vi "GUI Main Window.vi"() -> ()   [LabVIEW 2011]
doc: "Fast Orbit Feedback (FOFB) graphical user interface."
uses:
  Types Definitions/Type Configuration Loop Mode.ctl
  <vilib>/Platform/TimedLoop/XDataNode/timing_clust.ctl
  <vilib>/Platform/TimedLoop/XDataNode/nitl_modes.ctl
  <vilib>/Platform/TimedLoop/XDataNode/wakeup.ctl
  Types Definitions/Type Diagnostics Sample.ctl
  Types Definitions/Type Diagnostics Data.ctl
  Types Definitions/Type CPU Loads Array.ctl
  Types Definitions/Type CPU Loads.ctl
  Types Definitions/Type Monitoring Sample.ctl
  Types Definitions/Type FOFB Parameters.ctl
  Types Definitions/Type Network Configuration.ctl
  Types Definitions/Type FA Configuration.ctl
  Types Definitions/Type Response Matrix Measurement Configuration.ctl
  Types Definitions/Type Correction Algorithm Configuration.ctl
  Types Definitions/Type Acquisition Network Configuration.ctl
  Types Definitions/Type Actuation Network Configuration.ctl
  Types Definitions/Type BPM or PS Selector.ctl
  <vilib>/Analysis/5stat.llb/RMS (DBL).vi
  GUI Monitoring Graph Selection Window.vi
  <vilib>/Platform/TimedLoop/XDataNode/XDataNode.xnode
  <vilib>/Platform/TimedLoop/XDataNode/XDNodeRunTimeDep.lvlib
  File VIs.lvlib
  Type Definitions.lvlib
  Third Party/bean/bean.lvlib
  User Interface Window VIs.lvlib
  User Interface VIs.lvlib
  XML VIs.lvlib
  Filter VIs.lvlib
  <vilib>/Analysis/NI_AALPro.lvlib
panel:
  out "error out":errorcluster
  out "Connected":bool
  in  "Open Computer Performance":bool
  in  "Open BPM RMS/Min/Max Monitoring Graph":bool
  out "Orbit Path":path caption="Endereço da Órbita de Referência"
  in  "Open Configuration GUI":bool
  in  "Max Scale Y":dbl=1.0 min=0.001 max=20.0 format="%6.3g"
  in  "Max Scale X":dbl=1.0 min=0.001 max=20.0 format="%6.3g"
  in  "Auto-Scale":bool
  in  "Open BPM-PS Monitoring Graph":bool
  out "Reference Orbit":dbl[](array[numeric])
  in  "Orbit Source":enum32{"Zero", "From File", "Current Orbit"}(radio)
  out "Current Orbit":dbl[](array[numeric])
  out "Operation Mode (Controller to GUI)":T1(ring) caption="Modo de Operação"
  in  "Send Orbit":bool
  out "Min Y @":string="AMP05A" caption="@"
  out "MaxY @":string="AMP05A" caption="@"
  out "RMS Y":dbl=-1.1111 caption="RMS =" format="%#.4g"
  out "Min Y":dbl=-1.2564 caption="Min =" format="%#.4g"
  out "Max. Y":dbl=1.1111 caption="Max =" format="%#.4g"
  out "Min X @":string="AMP01A" caption="@"
  out "Max X @":string="AMP01A" caption="@"
  out "RMS X":dbl=21.1111 caption="RMS =" format="%#.4g"
  out "Min X":dbl=1.1111 caption="Min =" format="%#.4g"
  out "Max. X":dbl=1.1111 caption="Max =" format="%#.4g"
  out "Horizontal":cluster{i32, dbl}[](graph)
  out "Vertical":cluster{i32, dbl}[](graph)
  in  "Save Orbit":bool
  # "Órbita de Referência Local"
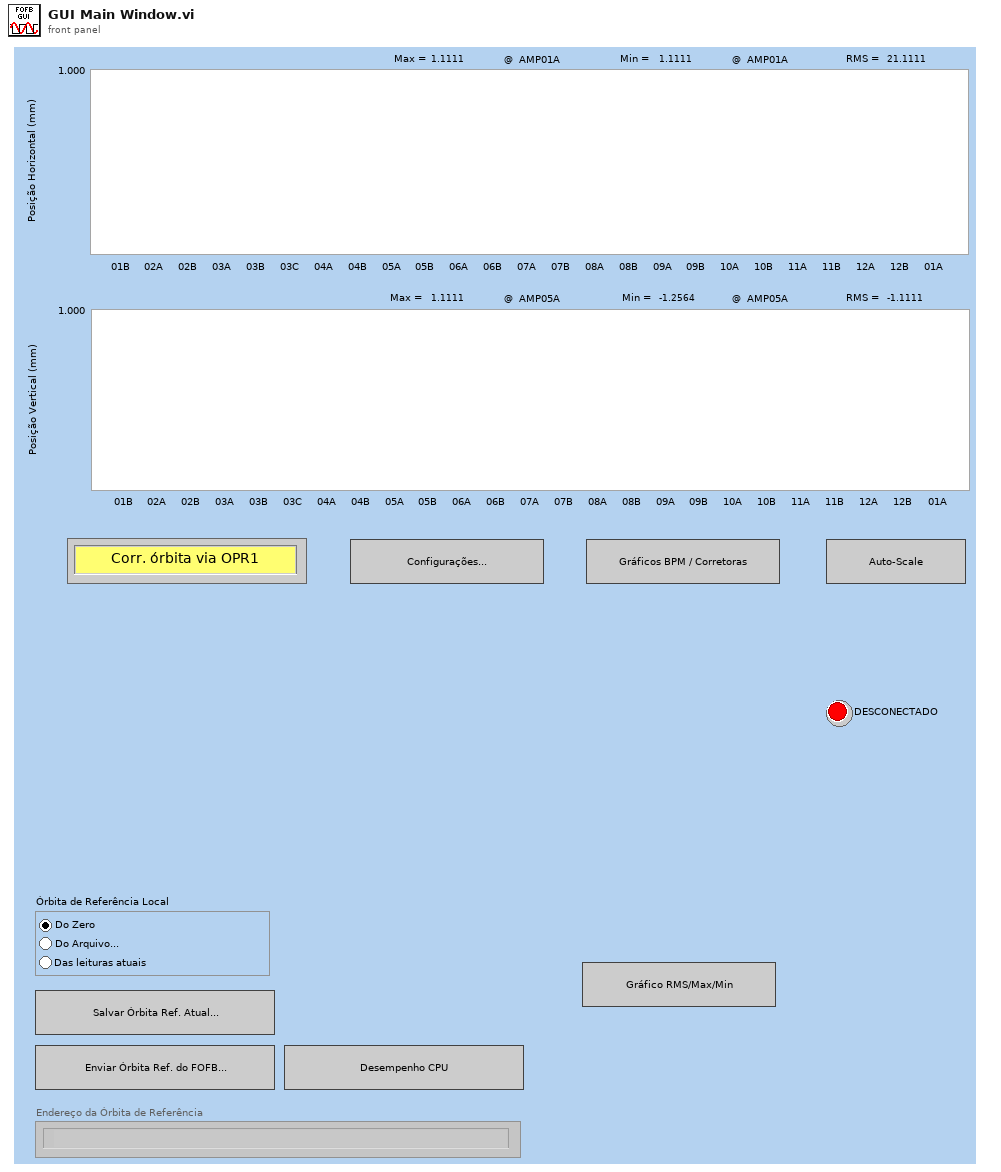
[diagram p1: front panel]
types:
  T1 = enum16{"Corr. órbita via OPR1", "Corr. órbita via FOFB", "Medida de Matriz Resposta"}
  T2 = enum8{"Enabled", "Disabled", "Disabled and Grayed Out"}
  T3 = typedef "Type Definitions.lvlib/Type Configuration Loop Mode.ctl" = enum8{"Operation Mode", "Request FOFB Parameters", "Send New FOFB Parameters", "Send Reference Orbit", "Request Response Matrix List Folder"}
  T4 = typedef "XDNodeRunTimeDep.lvlib/timing_clust.ctl" = cluster{"Expected End [f-1]":u64, "Actual End [f-1]":u64, "Finished Late? [f-1]":bool, "Expected End [i-1]":u64, "Actual End [i-1]":u64, "Finished Late? [i-1]":bool, "Expected Start [i]":u64, "Actual Start [i]":u64, "Expected Start [f]":u64, "Actual Start [f]":u64, "Source Name":string, "Structure Name":string, "Period":i64, "Deadline":i64, "Offset":i64, "Start":i64, "Priority":i32, "Timeout":i32, "Mode":T5, "Wakeup Reason":T6, "Error":errorcluster, "Source Type":string, "Secondary Source Type":string, "Global End Time":u64, "Global Start Time":u64, "Frame Duration":u64, "Iteration Duration":u64, "Assigned CPU":i32, "I/O Scan Engine Mode":u32}
  T5 = typedef "XDNodeRunTimeDep.lvlib/nitl_modes.ctl" = enum32{"No Change", "Process missed periods, maintain original phase", "Discard missed periods, maintain original phase", "Process missed periods, ignore original phase", "Discard missed periods, ignore original phase"}
  T6 = typedef "XDNodeRunTimeDep.lvlib/wakeup.ctl" = enum32{"Normal", "Aborted", "Asynchronous wakeup", "Timing source error", "Timed loop error", "Timeout"}
  T7 = enum32{"Invalid", "Standard", "Closed", "Hidden", "Minimized", "Maximized"}
  T8 = typedef "Type Definitions.lvlib/Type BPM or PS Selector.ctl" = cluster{"Name":string, "Active":bool}
  T9 = typedef "Type Definitions.lvlib/Type Diagnostics Sample.ctl" = cluster{"Timestamp":timestamp, "Diagnostics Data":T10}
  T10 = typedef "Type Definitions.lvlib/Type Diagnostics Data.ctl" = cluster{"Time-Critical Loop Missed Iterations":u32, "Time-Critical Loop Execution Time (usec)":u32, "FA Buffer Usage":u32, "Available Memory (bytes)":u32, "CPU Loads Array":T11}
  T11 = typedef "Type Definitions.lvlib/Type CPU Loads Array.ctl" = T12[]
  T12 = typedef "Type Definitions.lvlib/Type CPU Loads.ctl" = cluster{"Total (%)":dbl, "Time Critical (%)":dbl, "Timed Structures (%)":dbl, "High (%)":dbl, "Above Normal (%)":dbl, "Normal (%)":dbl, "Background (%)":dbl, "Idle (%)":dbl, "ISR (%)":dbl}
  T13 = enum16{"open", "open or create", "create or replace", "create", "open (read-only)"}
  T14 = typedef "Type Definitions.lvlib/Type FOFB GUI.ctl" = cluster{"Response Matrix List Folder Notifier":refnum<notifier>, "Send Reference Orbit Notifier":refnum<notifier>, "FOFB Parameters Notifier":refnum<notifier>, "Configuration Loop Mode Notifier":refnum<notifier>, "Stop VIs Notifier":refnum<notifier>, "GUI Configuration Notifier":refnum<notifier>, "Monitoring Data Notifier":refnum<queue>, "Performance Monitoring Data Notifier":refnum<queue>, "BPM / PS Monitoring Data Notifiers":refnum<queue>[], "Load Orbit Notifier":refnum<notifier>, "RMS Monitoring Data Queue":refnum<queue>, "GUI-Controller Connected Queue":refnum<queue>}
  T15 = typedef "Type Definitions.lvlib/Type FOFB Parameters.ctl" = cluster{"Network":T16, "Fast Acquisition":T17, "Response Matrix Measurement":T18, "Correction Algorithm":T19, "Acquisition Network":T20, "Actuation Network":T21}
  T16 = typedef "Type Definitions.lvlib/Type Network Configuration.ctl" = cluster{"FOFB Controller IP":string, "LNLS Control Network IP":string, "LNLS Control Network Power Supplies TCP Port":u16, "LNLS Control Network FOFB Configuration TCP Port":u16, "Data Server TCP Port":u16, "Monitoring Data TCP Port":u16, "Configuration GUI TCP Port":u16, "TCP Listening Timeout":i32}
  T17 = typedef "Type Definitions.lvlib/Type FA Configuration.ctl" = cluster{"Acquisition Period":u32, "Data Buffer Size":u32, "Monitoring Period":u32}
  T18 = typedef "Type Definitions.lvlib/Type Response Matrix Measurement Configuration.ctl" = cluster{"Step Amplitude":dbl, "Time Between Steps":u32, "Step Duration":u32, "Number of Averages":u32}
  T19 = typedef "Type Definitions.lvlib/Type Correction Algorithm Configuration.ctl" = cluster{"Correction Period":u32, "Reference Orbit Path":path, "Response Matrix Path":path, "Correction Matrix Path":path, "Horizontal Correction Factor":dbl, "Vertical Correction Factor":dbl, "Beam Current FOFB Threshold":dbl, "Decouple H-V":bool, "Use Additional BPM LPF":bool, "BPM LPF Cutoff":dbl}
  T20 = typedef "Type Definitions.lvlib/Type Acquisition Network Configuration.ctl" = cluster{"Chassis Name":string, "Variables":cluster{"Variable Name":string, "Matrix Order":u32, "Location":dbl, "Plane":enum8{"H", "V"}, "On Correction":bool}[]}[]
  T21 = typedef "Type Definitions.lvlib/Type Actuation Network Configuration.ctl" = cluster{"Chassis Name":string, "Variables":cluster{"Variable Name":string, "Matrix Order":u32, "RMM Step Factor":dbl, "Plane":enum8{"H", "V"}, "On Correction":bool, "Kc":dbl, "Ti":dbl, "Td":dbl}[]}[]
  T22 = typedef "Type Definitions.lvlib/Type Monitoring Sample.ctl" = cluster{"Timestamp":timestamp, "Sample":dbl[]}
  T23 = typedef "Type Definitions.lvlib/Type Monitoring Data.ctl" = cluster{"Timestamp":timestamp, "BPM Readings":dbl[], "PS Readings":dbl[], "PS FOFB Setpoints":dbl[], "PS Status per Rack":u8[], "PS ON-OFF per Rack":u8[], "Operation Mode":enum16{"Idle Mode", "Error Mode", "Manual Mode", "FOFB Mode", "RMM Mode"}, "Diagnostics Data":T10, "Controller Status Table":i32[]}
  T24 = enum16{"Idle Mode", "Error Mode", "Manual Mode", "FOFB Mode", "RMM Mode"}
  T25 = typedef "LVDateTimeRec.ctl" = cluster{"fractional second":dbl, "second":i32, "minute":i32, "hour":i32, "day of month":i32, "month":i32, "year":i32, "day of week":i32, "day of year":i32, "DST":i32}
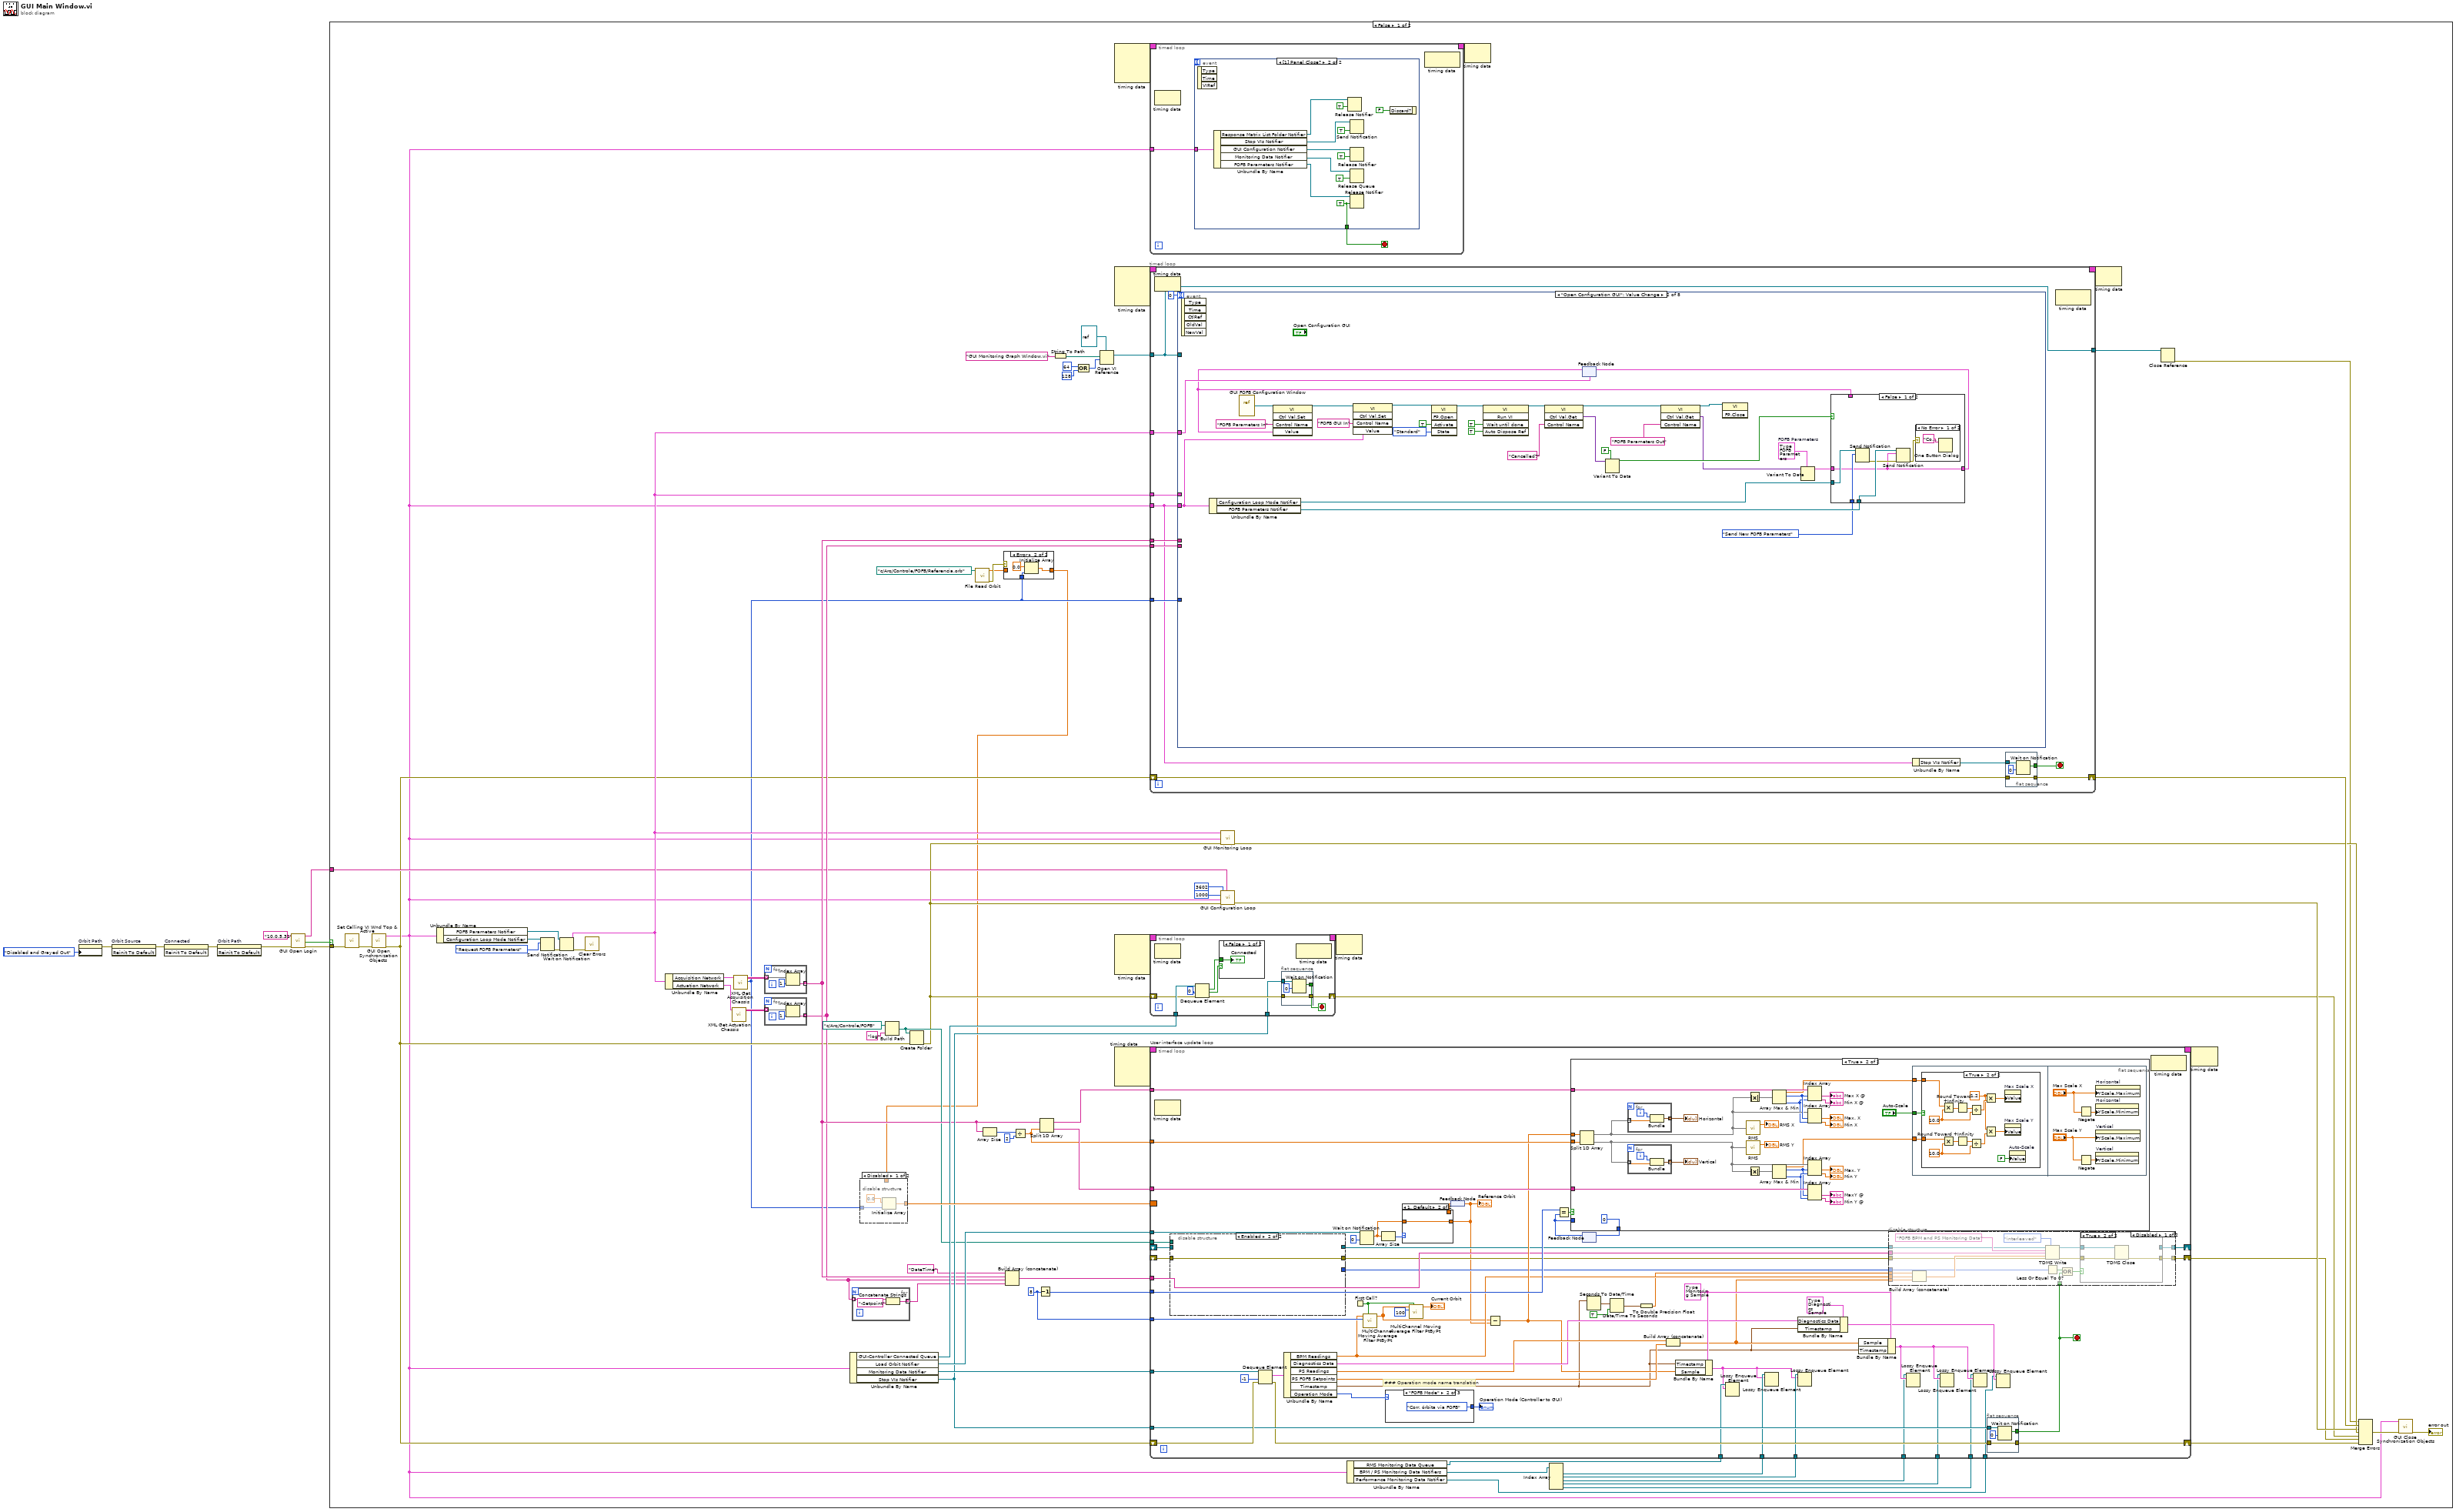
[diagram p0: block diagram]
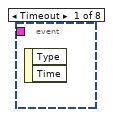
[diagram p5: hidden frame]
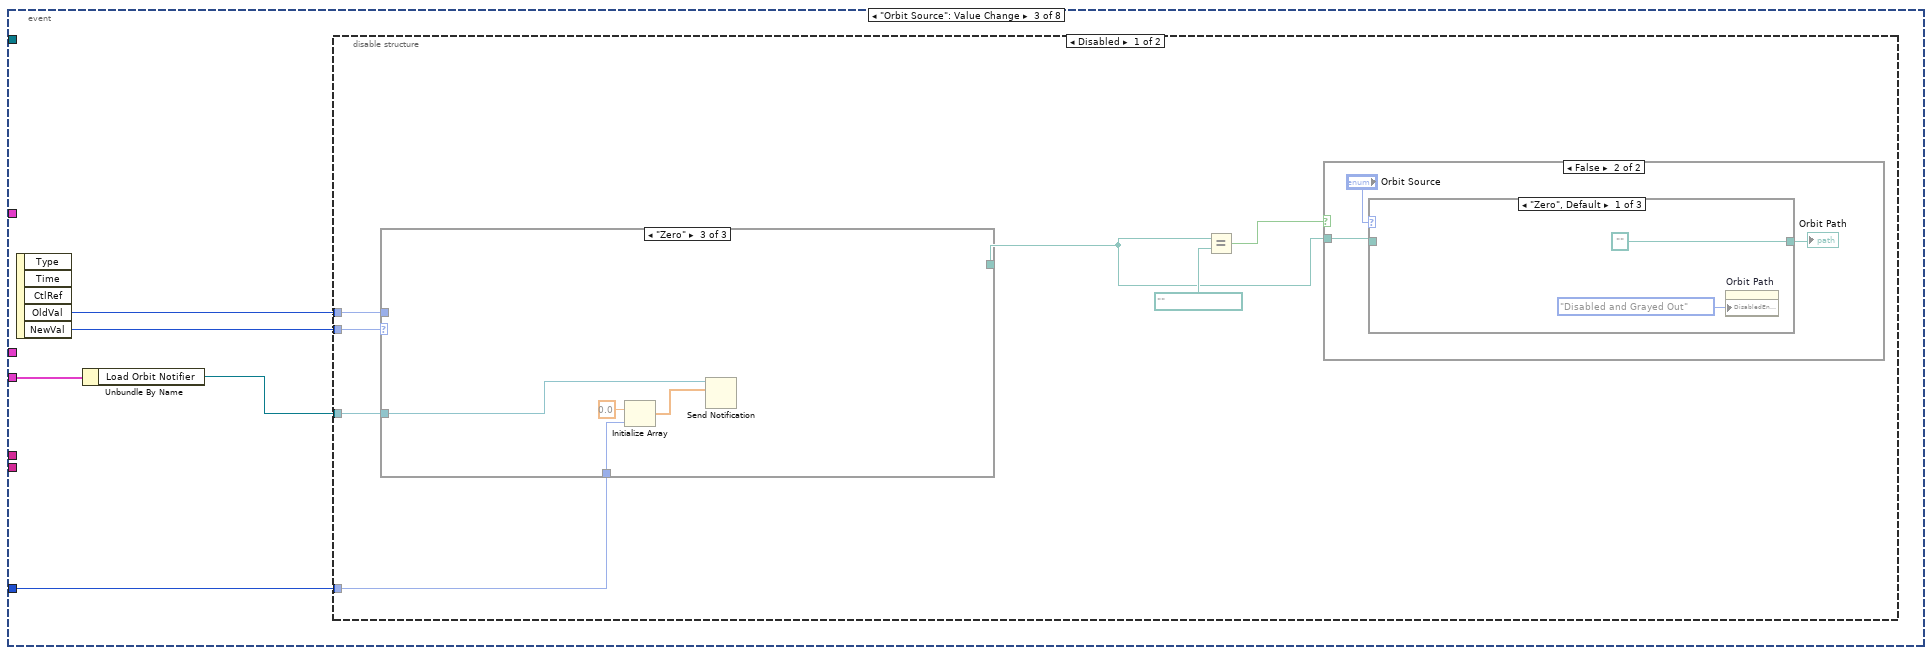
[diagram p8: hidden frame]
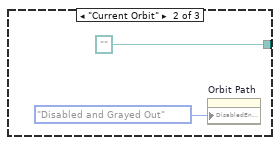
[diagram p10: hidden frame]
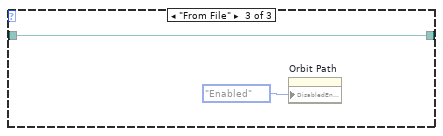
[diagram p11: hidden frame]
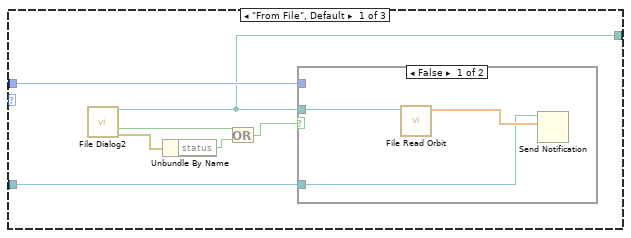
[diagram p12: hidden frame]
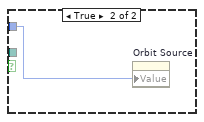
[diagram p13: hidden frame]
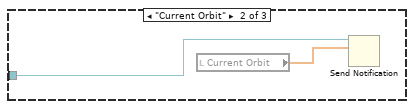
[diagram p14: hidden frame]
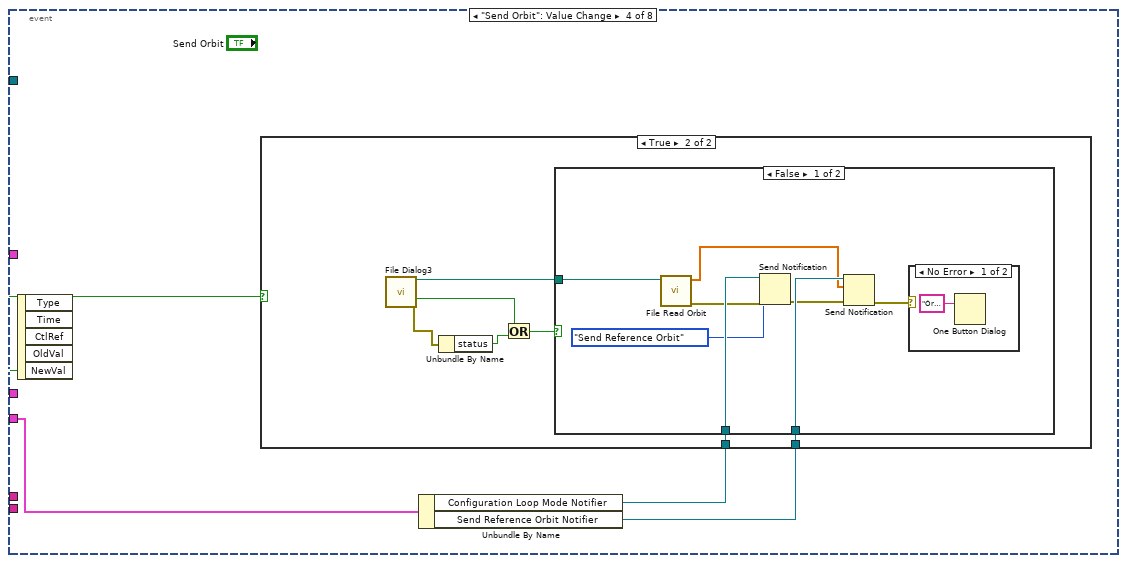
[diagram p16: hidden frame]
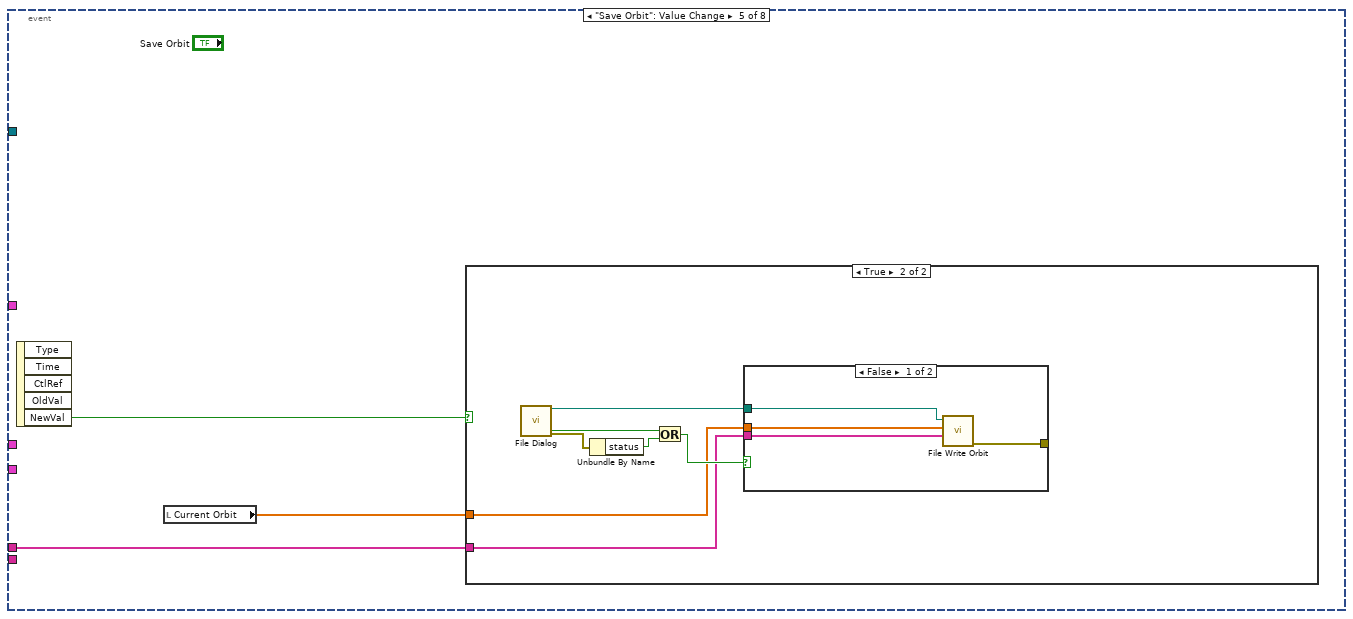
[diagram p20: hidden frame]
diagram:
  (unwired) T2."Disabled and Grayed Out" ("Disabled")
  n1 = property on="Orbit Path" class="Path"("DisabledEnum"=T2."Disabled and Grayed Out" ("Disabled")) -> (error out=w8:errorcluster)  [unwired: 2 in, 1 out]
  n2 = invoke on="Orbit Source" class="RadioBtnsControl (strict)" method="Reinit To Default"(error in=w8) -> (error out=w7:errorcluster)  [unwired: 2 in, 2 out]
  n3 = invoke on="Connected" class="Bool (strict)" method="Reinit To Default"(error in=w7) -> (error out=w6:errorcluster)  [unwired: 2 in, 2 out]
  n4 = invoke on="Orbit Path" class="Path" method="Reinit To Default"(error in=w6) -> (error out=w5:errorcluster)  [unwired: 2 in, 2 out]
  n5 = call "GUI Open Login.vi"("error in (no error)"=w5, "Controller IP Address in"="10.0.5.31" ("FOFB-Controller IP Address in")) -> ("error out"=w2:errorcluster, "Cancelled?"=w1:bool, "Controller IP Address out"=w3:string)  [unwired: 6 in, 1 out]
  n6 = case shown="False" w1 {
    tunnel: w2 -> [w20 _]
    tunnel: w3 -> [w21 _]
    frame False {
      w67 = u32 8 ("Number of Averages")
      n7 = call "Set Calling VI Wnd Top & Active.vi"("Error In"=w20) -> ("Error Out"=w19:errorcluster)  [unwired: 10 in]
      n8 = call "GUI Open Synchronization Objects.vi"("error in (no error)"=w19) -> ("error out"=w17:errorcluster, "FOFB GUI"=w11:T14)  [unwired: 9 in]
      n9 = Unbundle By Name(w11) -> ("FOFB Parameters Notifier"=w27:refnum<notifier>, "Configuration Loop Mode Notifier"=w28:refnum<notifier>)
      n10 = Send Notification(notification=Type_Configuration_Loop_Mode."Request FOFB Parameters", notifier=w28) -> (error out=w31:errorcluster)  [unwired: 1 in, 1 out]
      n11 = Wait on Notification(notifier=w27, error in (no error)=w31) -> (notification=w22:T15, error out=w25:errorcluster)  [unwired: 2 in, 2 out]
      n12 = call <vilib>:"Clear Errors.vi"("error in (no error)"=w25) -> ()  [unwired: 6 in, 1 out]
      n13 = Unbundle By Name(w22) -> ("Acquisition Network"=w77:T20, "Actuation Network"=w76:T21)
      n14 = call "XML Get Actuation Chassis.vi"("Actuation Network"=w76) -> ("Actuation Variable Names"=w74:string[][])  [unwired: 3 in, 7 out]
      n15 = call "XML Get Acquisition Chassis.vi"("Acquisition Network"=w77) -> ("Number of BPM Readings"=w12:i32, "Acquisition Variable Names"=w75:string[][])  [unwired: 4 in, 5 out]
      n16 = for {
        tunnel: w75 -> [w558] mode=indexing
        tunnel: [w557] -> w39 mode=indexing
        n17 = Index Array(array=w558, index=1) -> (element=w557:string)
      }
      n18 = for {
        tunnel: w74 -> [w555] mode=indexing
        tunnel: [w554] -> w37 mode=indexing
        n19 = Index Array(array=w555, index=1) -> (element=w554:string)
      }
      n20 = Unbundle By Name(w11) -> ("GUI-Controller Connected Queue"=w57:refnum<queue>, "Load Orbit Notifier"=w62:refnum<notifier>, "Monitoring Data Notifier"=w63:refnum<queue>, "Stop VIs Notifier"=w56:refnum<notifier>)
      n21 = for {
        tunnel: w37 -> [w96] mode=indexing
        tunnel: [w95] -> w36 mode=indexing
        n22 = Concatenate Strings(w96, "-Setpoint" ("string")) -> (w95:string)
      }
      n23 = Build Path(base path=path "c:/Arq/Controle/FOFB", name or relative path="log") -> (appended path=w32:path)
      n24 = Create Folder(path (use dialog)=w32, error in=w17) -> (error out=w16:errorcluster)  [unwired: 1 in, 2 out]
      n25 = call "File Read Orbit.vi"("file path (dialog if empty)"=path "c:/Arq/Controle/FOFB/Referencia.orb") -> ("error out"=w14:errorcluster, "Orbit"=w13:dbl[])  [unwired: 8 in, 1 out]
      n26 = Array Size(array=w39) -> (size(s)=w69:i32)
      n27 = case shown="Error" w14 {
        tunnel: w13 -> [w90 _]
        tunnel: [w90 w92] -> w10
        tunnel: w12 -> [_ w91]
        frame No Error {
        }
        frame Error {
          n28 = Initialize Array(0.0 ("element"), w91) -> (w92:dbl[])
        }
      }
      n29 = disable-structure shown="Disabled" {
        disable-tunnel: [w87 w89] -> w65
        disable-tunnel: w12 -> [w86 _]
        disable-tunnel: w10 -> [_ w89]
        frame Disabled {
          n30 = Initialize Array(0.0 ("element"), w86) -> (w87:dbl[])
        }
        frame Enabled {
        }
      }
      n31 = Build Array (concatenate)("DateTime" ("name or relative path"), w39, w37, w36) -> (w38:string[])
      n32 = Divide(x=w69, y=2) -> (x/y=w53:dbl)
      n33 = Decrement(x=w67) -> (x-1=w66:u32)
      n34 = Split 1D Array(array=w39, index=w53) -> (first subarray=w55:string[], second subarray=w54:string[])
      n35 = String To Path(string="GUI Monitoring Graph Window.vi") -> (path=w41:path)
      n36 = Compound Arithmetic op=OR(64 ("options"), 128 ("options")) -> (w45:i32)
      n37 = Open VI Reference(type specifier VI Refnum (for type only)=refnum<vi> refnum, vi path=w41, options=w45) -> (vi reference=w64:refnum<vi>)  [unwired: 3 in, 1 out]
      n38 = node-c288() -> (w85:T4)  [unwired: 4 in]
      n39 = node-c288() -> (w81:T4)  [unwired: 4 in]
      n40 = node-c288() -> (w79:T4)  [unwired: 4 in]
      n41 = node-c288() -> (w83:T4)  [unwired: 4 in]
      n42 = timed-loop {
        timing: w85 -> [_]
        timing-out: [_] -> w84
        tunnel: w11 -> [w561]
        stop <- w560 stop-if-true
        n43 = node-c288() -> ()  [unwired: 1 in, 1 out]
        n44 = event shown="[1] Panel Close?" {
          selector: _ -> [_ _]
          dyn-events: _ -> [_ _]
          timeout: _ -> [_ _]
          tunnel: w561 -> [_ w565]
          tunnel: [_ w566] -> w560
          event Timeout {
            n45 = event-data() -> ()  [unwired: 1 in, 2 out]
          }
          event Panel Close? {
            w566 = TRUE ("force destroy? (F)")
            n46 = event-data() -> ()  [unwired: 1 in, 3 out]
            n47 = Unbundle By Name(w565) -> ("Response Matrix List Folder Notifier"=w563:refnum<notifier>, "Stop VIs Notifier"=w570:refnum<notifier>, "GUI Configuration Notifier"=w572:refnum<notifier>, "Monitoring Data Notifier"=w567:refnum<queue>, "FOFB Parameters Notifier"=w573:refnum<notifier>)
            n48 = Release Notifier(notifier=w563, force destroy? (F)=TRUE) -> ()  [unwired: 1 in, 3 out]
            n49 = Send Notification(notification=TRUE, notifier=w570) -> ()  [unwired: 1 in, 2 out]
            n50 = Release Notifier(notifier=w572, force destroy? (F)=TRUE) -> ()  [unwired: 1 in, 3 out]
            n51 = Release Queue(queue=w567, force destroy? (F)=TRUE) -> ()  [unwired: 1 in, 3 out]
            n52 = Release Notifier(notifier=w573, force destroy? (F)=w566) -> ()  [unwired: 1 in, 3 out]
            n53 = event-data("Discard?"=FALSE) -> ()  [unwired: 1 in, 1 out]
          }
        }
        n54 = node-c288() -> ()  [unwired: 1 in, 1 out]
      }
      n55 = timed-loop {
        tunnel: w39 -> [w126]
        tunnel: w12 -> [w125]
        tunnel: w37 -> [w124]
        timing: w81 -> [_]
        timing-out: [_] -> w80
        tunnel: w64 -> [w123]
        tunnel: [w123] -> w60
        shift-right: [w120] -> w73
        shift-left: w17 -> [w121]
        tunnel: w11 -> [w118]
        tunnel: w22 -> [w122]
        tunnel: w22 -> [w115]
        stop <- w119 stop-if-true
        n56 = node-c288() -> ()  [unwired: 1 in, 1 out]
        n57 = event shown="[1] \"Open Configuration GUI\": Value Change" {
          selector: _ -> [_ _ _ _ _ _ _ _]
          dyn-events: _ -> [_ _ _ _ _ _ _ _]
          timeout: 0 -> [_ _ _ _ _ _ _ _]
          tunnel: w126 -> [_ _ _ _ w228 _ w253 _]
          tunnel: w125 -> [_ _ w171 _ _ _ _ _]
          tunnel: w124 -> [_ _ _ _ _ _ w255 _]
          tunnel: w123 -> [_ _ _ _ _ _ w254 _]
          tunnel: w118 -> [_ w136 w169 w209 _ _ _ _]
          tunnel: w122 -> [_ _ _ _ _ _ _ _]
          tunnel: w115 -> [_ w134 _ _ _ _ _ _]
          event Timeout {
            n58 = event-data() -> ()  [unwired: 1 in, 2 out]
          }
          event "Open Configuration GUI": Value Change {
            w144 = T15 {"Network"={"FOFB Controller IP"="", "LNLS Control Network IP"="", "LNLS Control Network Power Supplies TCP Port"=0, "LNLS Control Network FOFB Configuration TCP Port"=0, "Data Server TCP Port"=0, "Monitoring Data TCP Port"=0, "Configuration GUI TCP Port"=0, "TCP Listening Timeout"=0}, "Fast Acquisition"={"Acquisition Period"=0, "Data Buffer Size"=0, "Monitoring Period"=0}, "Response Matrix Measurement"={"Step Amplitude"=0.0, "Time Between Steps"=0, "Step Duration"=0, "Number of Averages"=0}, "Correction Algorithm"={"Correction Period"=0, "Reference Orbit Path"=path "", "Response Matrix Path"=path "", "Correction Matrix Path"=path "", "Horizontal Correction Factor"=0.0, "Vertical Correction Factor"=0.0, "Beam Current FOFB Threshold"=0.0, "Decouple H-V"=FALSE, "Use Additional BPM LPF"=FALSE, "BPM LPF Cutoff"=0.0}, "Acquisition Network"=[], "Actuation Network"=[]}  # FOFB Parameters
            n59 = event-data() -> ()  [unwired: 1 in, 5 out]
            n60 = Unbundle By Name(w136) -> ("Configuration Loop Mode Notifier"=w137:refnum<notifier>, "FOFB Parameters Notifier"=w143:refnum<notifier>)
            n61 = vi-ref "GUI FOFB Configuration Window.vi"() -> (w149:refnum<vi>)
            n62 = feedback #1(w134) -> (w133:T15)
            n63 = invoke class="VI" method="Ctrl Val.Set"(reference=w149, "Control Name"="FOFB Parameters In", "Value"=w133) -> (reference out=w140:refnum<vi>)  [unwired: 2 in, 4 out]
            n64 = invoke class="VI" method="Ctrl Val.Set"(reference=w140, "Control Name"="FOFB GUI In", "Value"=w136) -> (reference out=w139:refnum<vi>)  [unwired: 2 in, 4 out]
            n65 = invoke class="VI" method="FP.Open"(reference=w139, "Activate"=TRUE ("Activate?"), "State"=T7."Standard") -> (reference out=w156:refnum<vi>)  [unwired: 2 in, 4 out]
            n66 = invoke class="VI" method="Run VI"(reference=w156, "Wait until done"=TRUE ("Wait Until Done"), "Auto Dispose Ref"=TRUE ("Auto Dispose Reference")) -> (reference out=w157:refnum<vi>)  [unwired: 2 in, 4 out]
            n67 = invoke class="VI" method="Ctrl Val.Get"(reference=w157, "Control Name"="Cancelled?") -> (reference out=w148:refnum<vi>, "Get Control Value Variant"=w151:variant)  [unwired: 2 in, 2 out]
            n68 = Variant To Data(type=FALSE ("Stop?"), Variant=w151) -> (data=w150:bool)  [unwired: 1 in, 1 out]
            n69 = invoke class="VI" method="Ctrl Val.Get"(reference=w148, "Control Name"="FOFB Parameters Out") -> (reference out=w147:refnum<vi>, "Get Control Value Variant"=w145:variant)  [unwired: 2 in, 2 out]
            n70 = invoke class="VI" method="FP.Close"(reference=w147) -> ()  [unwired: 2 in, 3 out]
            n71 = Variant To Data(type=w144, Variant=w145) -> (data=w142:T15)  [unwired: 1 in, 1 out]
            n72 = case shown="False" w150 {
              tunnel: w137 -> [w166 _]
              tunnel: w143 -> [w165 _]
              tunnel: w142 -> [w162 _]
              tunnel: [w162 w168] -> w135
              tunnel: Type_Configuration_Loop_Mode."Send New FOFB Parameters" ("notification") -> [w163 _]
              tunnel: w133 -> [_ w168]
              frame False {
                n73 = Send Notification(notification=w163, notifier=w166) -> (error out=w164:errorcluster)  [unwired: 1 in, 1 out]
                n74 = Send Notification(notification=w162, notifier=w165, error in (no error)=w164) -> (error out=w161:errorcluster)  [unwired: 1 out]
                n75 = case shown="No Error" w161 {
                  frame No Error {
                    n76 = One Button Dialog(message="Configurações alteradas com sucesso") -> ()  [unwired: 1 in, 1 out]
                  }
                  frame Error {
                  }
                }
              }
              frame True {
              }
            }
            n77 = feedback-in #1(w135) -> ()
          }
          event "Orbit Source": Value Change {
            n78 = event-data() -> ("OldVal"=w172:enum32{"Zero", "From File", "Current Orbit"}, "NewVal"=w173:enum32{"Zero", "From File", "Current Orbit"})  [unwired: 1 in, 3 out]
            n79 = Unbundle By Name(w169) -> ("Load Orbit Notifier"=w170:refnum<notifier>)
            n80 = disable-structure shown="Disabled" {
              disable-tunnel: w173 -> [w180 _]
              disable-tunnel: w172 -> [w179 _]
              disable-tunnel: w171 -> [w178 _]
              disable-tunnel: w170 -> [w174 _]
              frame Disabled {
                n81 = case shown="\"Zero\"" w180 {
                  tunnel: w174 -> [w193 w202 w206]
                  tunnel: w179 -> [w192 _ _]
                  tunnel: w178 -> [_ _ w205]
                  tunnel: [w191 _ _] -> w176
                  frame "From File", Default {
                    n82 = call "File Dialog2"() -> ("selected path"=w191:path, "cancelled"=w190:bool, "error out"=w194:errorcluster)  [unwired: 12 in, 1 out]
                    n83 = Unbundle By Name(w194) -> ("status"=w195:bool)
                    n84 = Or(x=w190, y=w195) -> (x .or. y?=w196:bool)
                    n85 = case shown="False" w196 {
                      tunnel: w191 -> [w199 _]
                      tunnel: w193 -> [w197 _]
                      tunnel: w192 -> [_ w200]
                      frame False {
                        n86 = call "File Read Orbit.vi"("file path (dialog if empty)"=w199) -> ("Orbit"=w198:dbl[])  [unwired: 8 in, 2 out]
                        n87 = Send Notification(notification=w198, notifier=w197) -> ()  [unwired: 1 in, 2 out]
                      }
                      frame True {
                        n88 = property on="Orbit Source" class="RadioBtnsControl (strict)"("Value"=w200) -> ()  [unwired: 2 in, 2 out]
                      }
                    }
                  }
                  frame "Current Orbit" {
                    n89 = local read "Current Orbit"() -> (w201:dbl[])
                    n90 = Send Notification(notification=w201, notifier=w202) -> ()  [unwired: 1 in, 2 out]
                  }
                  frame "Zero" {
                    n91 = Initialize Array(0.0 ("element"), w205) -> (w204:dbl[])
                    n92 = Send Notification(notification=w204, notifier=w206) -> ()  [unwired: 1 in, 2 out]
                  }
                }
                n93 = Equal?(x=w176, y=path "" ("Orbit Path")) -> (x = y?=w175:bool)
                n94 = case shown="False" w175 {
                  tunnel: w176 -> [_ w181]
                  frame True {
                  }
                  frame False {
                    n95 = case shown="\"Zero\", Default" "Orbit Source" {
                      tunnel: w181 -> [_ _ w189]
                      tunnel: [path "" ("selected path") path "" ("selected path") w189] -> w183
                      frame "Zero", Default {
                        n96 = property on="Orbit Path" class="Path"("DisabledEnum"=T2."Disabled and Grayed Out" ("Disabled")) -> ()  [unwired: 2 in, 2 out]
                      }
                      frame "Current Orbit" {
                        n97 = property on="Orbit Path" class="Path"("DisabledEnum"=T2."Disabled and Grayed Out" ("Disabled")) -> ()  [unwired: 2 in, 2 out]
                      }
                      frame "From File" {
                        n98 = property on="Orbit Path" class="Path"("DisabledEnum"=T2."Enabled" ("Disabled")) -> ()  [unwired: 2 in, 2 out]
                      }
                    }
                    "Orbit Path" <- w183
                  }
                }
              }
              frame Enabled {
              }
            }
          }
          event "Send Orbit": Value Change {
            n99 = event-data() -> ("NewVal"=w210:bool)  [unwired: 1 in, 4 out]
            n100 = Unbundle By Name(w209) -> ("Configuration Loop Mode Notifier"=w208:refnum<notifier>, "Send Reference Orbit Notifier"=w207:refnum<notifier>)
            n101 = case shown="True" w210 {
              tunnel: w208 -> [_ w212]
              tunnel: w207 -> [_ w211]
              frame False {
              }
              frame True {
                n102 = call "File Dialog3"() -> ("selected path"=w213:path, "cancelled"=w217:bool, "error out"=w215:errorcluster)  [unwired: 12 in, 1 out]
                n103 = Unbundle By Name(w215) -> ("status"=w216:bool)
                n104 = Or(x=w217, y=w216) -> (x .or. y?=w214:bool)
                n105 = case shown="False" w214 {
                  tunnel: w213 -> [w225 _]
                  tunnel: w212 -> [w224 _]
                  tunnel: w211 -> [w223 _]
                  frame False {
                    n106 = call "File Read Orbit.vi"("file path (dialog if empty)"=w225) -> ("error out"=w222:errorcluster, "Orbit"=w219:dbl[])  [unwired: 8 in, 1 out]
                    n107 = Send Notification(notification=Type_Configuration_Loop_Mode."Send Reference Orbit", notifier=w224, error in (no error)=w222) -> (error out=w221:errorcluster)  [unwired: 1 out]
                    n108 = Send Notification(notification=w219, notifier=w223, error in (no error)=w221) -> (error out=w218:errorcluster)  [unwired: 1 out]
                    n109 = case shown="No Error" w218 {
                      frame No Error {
                        n110 = One Button Dialog(message="Órbita de referência alterada com sucesso") -> ()  [unwired: 1 in, 1 out]
                      }
                      frame Error {
                      }
                    }
                  }
                  frame True {
                  }
                }
              }
            }
          }
          event "Save Orbit": Value Change {
            n111 = event-data() -> ("NewVal"=w229:bool)  [unwired: 1 in, 4 out]
            n112 = local read "Current Orbit"() -> (w227:dbl[])
            n113 = case shown="True" w229 {
              tunnel: w228 -> [_ w231]
              tunnel: w227 -> [_ w230]
              frame False {
              }
              frame True {
                n114 = call "File Dialog"() -> ("selected path"=w232:path, "cancelled"=w234:bool, "error out"=w236:errorcluster)  [unwired: 12 in, 1 out]
                n115 = Unbundle By Name(w236) -> ("status"=w235:bool)
                n116 = Or(x=w234, y=w235) -> (x .or. y?=w233:bool)
                n117 = case shown="False" w233 {
                  tunnel: w232 -> [w240 _]
                  tunnel: w231 -> [w239 _]
                  tunnel: w230 -> [w238 _]
                  tunnel: [w237 _] -> _
                  frame False {
                    n118 = call "File Write Orbit.vi"("BPM Reading Names"=w239, "Orbit"=w238, "file path (dialog if empty)"=w240) -> ("error out"=w237:errorcluster)  [unwired: 7 in]
                  }
                  frame True {
                  }
                }
              }
            }
          }
          event "Open BPM RMS/Min/Max Monitoring Graph": Value Change {
            n119 = event-data() -> ("NewVal"=w241:bool)  [unwired: 1 in, 4 out]
            n120 = case shown="True" w241 {
              frame False {
              }
              frame True {
                n121 = vi-ref "GUI BPM RMS Min Max Monitoring Graph Window.vi"() -> (w246:refnum<vi>)
                n122 = invoke class="VI" method="FP.Open"(reference=w246, "Activate"=TRUE ("Activate?"), "State"=T7."Standard") -> (reference out=w245:refnum<vi>, error out=w243:errorcluster)  [unwired: 2 in, 3 out]
                n123 = call <vilib>:"Clear Errors.vi"("error in (no error)"=w243) -> ("error out"=w244:errorcluster)  [unwired: 6 in]
                n124 = invoke class="VI" method="Run VI"(reference=w245, error in=w244, "Wait until done"=FALSE ("Wait Until Done"), "Auto Dispose Ref"=FALSE ("Auto Dispose Reference")) -> (error out=w242:errorcluster)  [unwired: 1 in, 4 out]
                n125 = call <vilib>:"Clear Errors.vi"("error in (no error)"=w242) -> ()  [unwired: 6 in, 1 out]
              }
            }
          }
          event "Open BPM-PS Monitoring Graph": Value Change {
            n126 = event-data() -> ()  [unwired: 1 in, 5 out]
            n127 = vi-ref "User Interface Window VIs.lvlib:GUI Monitoring Graph Selection Window.vi"() -> (w252:refnum<vi>)
            n128 = invoke class="VI" method="FP.Open"(reference=w252, "Activate"=TRUE ("Activate?"), "State"=T7."Standard") -> (reference out=w251:refnum<vi>)  [unwired: 2 in, 4 out]
            n129 = invoke class="VI" method="Run VI"(reference=w251) -> (reference out=w261:refnum<vi>)  [unwired: 4 in, 4 out]
            n130 = invoke class="VI" method="Ctrl Val.Get"(reference=w261, "Control Name"="Graph Selector Out") -> (reference out=w256:refnum<vi>, "Get Control Value Variant"=w263:variant)  [unwired: 2 in, 2 out]
            n131 = Variant To Data(type=T8[] [{"Name"="", "Active"=FALSE}] ("BPM Graph Selector Horizontal"), Variant=w263) -> (data=w257:T8[])  [unwired: 1 in, 1 out]
            n132 = invoke class="VI" method="Ctrl Val.Get"(reference=w256, "Control Name"="Start plotting?") -> (reference out=w268:refnum<vi>, "Get Control Value Variant"=w259:variant)  [unwired: 2 in, 2 out]
            n133 = Variant To Data(type=TRUE, Variant=w259) -> (data=w258:bool)  [unwired: 1 in, 1 out]
            n134 = case shown="True" w258 {
              tunnel: w257 -> [_ w273]
              tunnel: w254 -> [_ w272]
              tunnel: w255 -> [_ w271]
              tunnel: w253 -> [_ w270]
              frame False {
              }
              frame True {
                n135 = for {
                  tunnel: w273 -> [w364] mode=indexing
                  tunnel: [w363] -> w269 mode=indexing
                  n136 = Unbundle By Name(w364) -> ("Active"=w363:bool)
                }
                n137 = for {
                  tunnel: w269 -> [w277] mode=indexing
                  tunnel: w272 -> [w278]
                  tunnel: w271 -> [w275]
                  tunnel: w270 -> [w274]
                  i -> [w276]
                  n138 = case shown="0, Default" w276 {
                    tunnel: w278 -> [w281 w297 w313 w330 w347]
                    tunnel: w277 -> [w280 w296 w312 w329 w346]
                    tunnel: w275 -> [w279 w295 w311 w328 w345]
                    tunnel: w274 -> [_ _ _ w327 w344]
                    frame 2 {
                      n139 = case shown="True" w280 {
                        tunnel: w281 -> [_ w291]
                        tunnel: w279 -> [_ w287]
                        frame False {
                        }
                        frame True {
                          n140 = call "GUI PS Group Indexes.vi"("PS Group"=enum16{"ACH", "ACV", "ALV"}."ACH") -> ("Indexes"=w283:i32[])  [unwired: 10 in]
                          n141 = call "GUI Build PS Vector.vi"("PS Indexes in"=w283) -> ("PS Indexes out"=w284:i32[])  [unwired: 10 in]
                          n142 = for {
                            tunnel: w287 -> [w292]
                            tunnel: w283 -> [w294] mode=indexing
                            tunnel: [w293] -> w286 mode=indexing
                            n143 = Index Array(array=w292, index=w294) -> (element=w293:string)
                          }
                          n144 = call-by-ref "Start Asynchronous Call"(reference=w291, "Graph Unit"="Corrente (A)", "Window Title"="FOFB - Gráfico Grupo ACH", "BPM?"=FALSE, "Monitoring Queue Name"="ACH Monitoring Data" ("Window Title"), "Selected Readings"=w284, "Variable Names"=w286) -> ()  [unwired: 7 in, 2 out]
                        }
                      }
                    }
                    frame 3 {
                      n145 = case shown="True" w296 {
                        tunnel: w297 -> [_ w307]
                        tunnel: w295 -> [_ w303]
                        frame False {
                        }
                        frame True {
                          n146 = call "GUI PS Group Indexes.vi"("PS Group"=enum16{"ACH", "ACV", "ALV"}."ACV") -> ("Indexes"=w298:i32[])  [unwired: 10 in]
                          n147 = call "GUI Build PS Vector.vi"("PS Indexes in"=w298) -> ("PS Indexes out"=w300:i32[])  [unwired: 10 in]
                          n148 = for {
                            tunnel: w303 -> [w308]
                            tunnel: w298 -> [w310] mode=indexing
                            tunnel: [w309] -> w302 mode=indexing
                            n149 = Index Array(array=w308, index=w310) -> (element=w309:string)
                          }
                          n150 = call-by-ref "Start Asynchronous Call"(reference=w307, "Graph Unit"="Corrente (A)", "Window Title"="FOFB - Gráfico Grupo ACV", "BPM?"=FALSE, "Monitoring Queue Name"="ACV Monitoring Data" ("Window Title"), "Selected Readings"=w300, "Variable Names"=w302) -> ()  [unwired: 7 in, 2 out]
                        }
                      }
                    }
                    frame 4 {
                      n151 = case shown="True" w312 {
                        tunnel: w313 -> [_ w323]
                        tunnel: w311 -> [_ w319]
                        frame False {
                        }
                        frame True {
                          n152 = call "GUI PS Group Indexes.vi"("PS Group"=enum16{"ACH", "ACV", "ALV"}."ALV") -> ("Indexes"=w315:i32[])  [unwired: 10 in]
                          n153 = call "GUI Build PS Vector.vi"("PS Indexes in"=w315) -> ("PS Indexes out"=w316:i32[])  [unwired: 10 in]
                          n154 = for {
                            tunnel: w319 -> [w324]
                            tunnel: w315 -> [w326] mode=indexing
                            tunnel: [w325] -> w318 mode=indexing
                            n155 = Index Array(array=w324, index=w326) -> (element=w325:string)
                          }
                          n156 = call-by-ref "Start Asynchronous Call"(reference=w323, "Graph Unit"="Corrente (A)", "Window Title"="FOFB - Gráfico Grupo ALV", "BPM?"=FALSE, "Monitoring Queue Name"="ALV Monitoring Data" ("Window Title"), "Selected Readings"=w316, "Variable Names"=w318) -> ()  [unwired: 7 in, 2 out]
                        }
                      }
                    }
                    frame 0, Default {
                      n157 = case shown="True" w329 {
                        tunnel: w330 -> [_ w339]
                        tunnel: w328 -> [_ _]
                        tunnel: w327 -> [_ w332]
                        frame False {
                        }
                        frame True {
                          n158 = for {
                            N: 25 -> [_]
                            tunnel: [w340] -> w333 mode=indexing
                            i -> [w340]
                          }
                          n159 = for {
                            tunnel: w332 -> [w341]
                            tunnel: w333 -> [w343] mode=indexing
                            tunnel: [w342] -> w335 mode=indexing
                            n160 = Index Array(array=w341, index=w343) -> (element=w342:string)
                          }
                          n161 = call-by-ref "Start Asynchronous Call"(reference=w339, "Graph Unit"="Amplitude (mm)", "Window Title"="FOFB - Gráfico BPMs Horizontais", "BPM?"=TRUE, "Monitoring Queue Name"="BPM Horizontal Monitoring Data" ("Window Title"), "Selected Readings"=w333, "Variable Names"=w335) -> ()  [unwired: 7 in, 2 out]
                        }
                      }
                    }
                    frame 1 {
                      n162 = case shown="True" w346 {
                        tunnel: w347 -> [_ w356]
                        tunnel: w345 -> [_ _]
                        tunnel: w344 -> [_ w349]
                        frame False {
                        }
                        frame True {
                          w351 = 25
                          n163 = for {
                            N: w351 -> [_]
                            tunnel: w351 -> [w359]
                            tunnel: [w357] -> w350 mode=indexing
                            i -> [w358]
                            n164 = Add(x=w359, y=w358) -> (x+y=w357:i32)
                          }
                          n165 = for {
                            tunnel: w349 -> [w360]
                            tunnel: w350 -> [w362] mode=indexing
                            tunnel: [w361] -> w352 mode=indexing
                            n166 = Index Array(array=w360, index=w362) -> (element=w361:string)
                          }
                          n167 = call-by-ref "Start Asynchronous Call"(reference=w356, "Graph Unit"="Amplitude (mm)", "Window Title"="FOFB - Gráfico BPMs Verticais", "BPM?"=TRUE, "Monitoring Queue Name"="BPM Vertical Monitoring Data" ("Window Title"), "Selected Readings"=w350, "Variable Names"=w352) -> ()  [unwired: 7 in, 2 out]
                        }
                      }
                    }
                  }
                }
              }
            }
            n168 = invoke class="VI" method="FP.Close"(reference=w268) -> ()  [unwired: 2 in, 3 out]
          }
          event "Open Computer Performance": Value Change {
            n169 = event-data() -> ("NewVal"=w365:bool)  [unwired: 1 in, 4 out]
            n170 = case shown="True" w365 {
              frame False {
              }
              frame True {
                n171 = vi-ref "GUI Controller Performace Window.vi"() -> (w372:refnum<vi>)
                n172 = invoke class="VI" method="FP.Open"(reference=w372, "Activate"=TRUE ("Activate?"), "State"=T7."Standard") -> (reference out=w366:refnum<vi>, error out=w371:errorcluster)  [unwired: 2 in, 3 out]
                n173 = call <vilib>:"Clear Errors.vi"("error in (no error)"=w371) -> ("error out"=w368:errorcluster)  [unwired: 6 in]
                n174 = invoke class="VI" method="Run VI"(reference=w366, error in=w368, "Wait until done"=FALSE ("Wait Until Done"), "Auto Dispose Ref"=FALSE ("Auto Dispose Reference")) -> (error out=w367:errorcluster)  [unwired: 1 in, 4 out]
                n175 = call <vilib>:"Clear Errors.vi"("error in (no error)"=w367) -> ()  [unwired: 6 in, 1 out]
              }
            }
          }
        }
        n176 = Unbundle By Name(w118) -> ("Stop VIs Notifier"=w117:refnum<notifier>)
        n177 = flat-sequence {
          tunnel: w121 -> [w127]
          tunnel: w117 -> [w130]
          tunnel: [w129] -> w119
          tunnel: [w127] -> w120
          frame #0 {
            n178 = Wait on Notification(notifier=w130, timeout in ms (-1)=0) -> (notification=w129:bool)  [unwired: 2 in, 3 out]
          }
        }
        n179 = node-c288() -> ()  [unwired: 1 in, 1 out]
      }
      n180 = timed-loop {
        timing: w79 -> [_]
        timing-out: [_] -> w78
        tunnel: w57 -> [w102]
        tunnel: w56 -> [w99]
        shift-right: [w98] -> w26
        shift-left: w16 -> [w97]
        stop <- w101 stop-if-true
        n181 = node-c288() -> ()  [unwired: 1 in, 1 out]
        n182 = Dequeue Element(queue=w102, timeout in ms (-1)=0, error in (no error)=w97) -> (element=w105:bool, timed out?=w104:bool, error out=w100:errorcluster)  [unwired: 1 out]
        n183 = case shown="False" w104 {
          tunnel: w105 -> [w110 _]
          frame False {
            "Connected" <- w110
          }
          frame True {
          }
        }
        n184 = flat-sequence {
          tunnel: [w109] -> w98
          tunnel: w100 -> [w109]
          tunnel: w99 -> [w108]
          tunnel: [w107] -> w101
          frame #0 {
            n185 = Wait on Notification(notifier=w108, timeout in ms (-1)=0) -> (notification=w107:bool)  [unwired: 2 in, 3 out]
          }
        }
        n186 = node-c288() -> ()  [unwired: 1 in, 1 out]
      }
      n187 = call "GUI Monitoring Loop.vi"("error in (no error)"=w16, "Sync Objects"=w11, "FOFB Parameters"=w22) -> ("error out"=w71:errorcluster)  [unwired: 8 in]
      n188 = call "GUI Configuration Loop.vi"("FOFB Controller IP"=w21, "error in (no error)"=w16, "FOFB GUI"=w11, "TCP Listening Timeout"=1000 ("timeout ms (60000)"), "Configuration GUI TCP Port"=u16 3602 ("remote port or service name")) -> ("error out"=w70:errorcluster)  [unwired: 6 in]
      n189 = node-c288(w78) -> ()  [unwired: 1 out]
      n190 = Unbundle By Name(w11) -> ("RMS Monitoring Data Queue"=w61:refnum<queue>, "BPM / PS Monitoring Data Notifiers"=w52:refnum<queue>[], "Performance Monitoring Data Notifier"=w46:refnum<queue>)
      n191 = node-c288(w84) -> ()  [unwired: 1 out]
      n192 = Index Array(array=w52) -> (element #1=w51:refnum<queue>, element #2=w50:refnum<queue>, element #3=w49:refnum<queue>, element #4=w48:refnum<queue>, element #5=w47:refnum<queue>)  [unwired: 5 in]
      n193 = timed-loop "User interface update loop" {
        tunnel: w63 -> [w436]
        shift-right: [w424] -> w72
        shift-left: w17 -> [w435]
        border: w65 -> [_]
        tunnel: w62 -> [w433]
        tunnel: w67 -> [w426]
        tunnel: w66 -> [w425]
        tunnel: w56 -> [w423]
        tunnel: w61 -> [w420]
        timing: w83 -> [_]
        timing-out: [_] -> w82
        tunnel: w55 -> [w415]
        tunnel: w54 -> [w414]
        tunnel: w53 -> [w413]
        tunnel: w51 -> [w406]
        tunnel: w50 -> [w405]
        tunnel: w49 -> [w404]
        tunnel: w48 -> [w403]
        tunnel: w47 -> [w402]
        tunnel: w46 -> [w401]
        tunnel: w38 -> [w394]
        shift-right: [w381] -> w33
        shift-left: _ -> [w384]
        shift-right: [w382] -> _
        shift-left: _ -> [w386]
        tunnel: w32 -> [w383]
        stop <- w379 stop-if-true
        w409 = T22 {"Timestamp"=timestamp(0 s since 1904-01-01), "Sample"=[]} ("Monitoring Sample")
        # "### Operation mode name translation"
        n194 = node-c288() -> ()  [unwired: 1 in, 1 out]
        n195 = disable-structure shown="Enabled" {
          disable-tunnel: [w445 _] -> w387
          disable-tunnel: w386 -> [w444 _]
          disable-tunnel: [w443 w461] -> w385
          disable-tunnel: w384 -> [w442 w461]
          disable-tunnel: w383 -> [w441 _]
          disable-tunnel: [w437 _] -> w380
          frame Disabled {
            n196 = feedback #2(u32 0 ("Number of Averages")) -> (w439:u32)
            n197 = Less Or Equal To 0?(x=w439) -> (x <= 0?=w438:bool)
            n198 = case shown="True" w438 {
              tunnel: [w449 w458] -> w445
              tunnel: w444 -> [w449 _]
              tunnel: [w448 w457] -> w443
              tunnel: w442 -> [w448 w456]
              tunnel: w441 -> [_ w451]
              tunnel: w439 -> [w447 _]
              tunnel: [w446 u32 12000 ("Number of Averages")] -> w437
              frame False {
                n199 = Decrement(x=w447) -> (x-1=w446:u32)
              }
              frame True {
                # "###"
                n200 = Get Date/Time In Seconds() -> (seconds since 1Jan1904=w454:timestamp)
                n201 = Format Date/Time String(time format string (%c)="%Y.%m.%d-%Hh%Mm%S%3u.tdms", seconds (now)=w454) -> (date/time string=w452:string)  [unwired: 1 in]
                n202 = Build Path(base path=w451, name or relative path=w452) -> (appended path=w460:path)
                n203 = TDMS Open(7:enum16{"1.0", "2.0"}."2.0" ("file format version (2.0)"), 8:w456, 10:T13."create or replace" ("operation (0:open)"), 11:w460) -> (0:w457:errorcluster, 3:w458:refnum<k34>)  [unwired: 2 in]
              }
            }
            n204 = feedback-in #2(w437) -> ()
          }
          frame Enabled {
          }
        }
        n205 = Dequeue Element(queue=w436, timeout in ms (-1)=-1, error in (no error)=w435) -> (element=w400:T23, error out=w421:errorcluster)  [unwired: 2 out]
        n206 = Unbundle By Name(w400) -> ("BPM Readings"=w393:dbl[], "Diagnostics Data"=w399:T10, "PS Readings"=w411:dbl[], "PS FOFB Setpoints"=w412:dbl[], "Timestamp"=w390:timestamp, "Operation Mode"=w398:T24)
        n207 = First Call?() -> (First Call?: T/F=w416:bool)
        n208 = Wait on Notification(notifier=w433, timeout in ms (-1)=0) -> (notification=w430:dbl[])  [unwired: 2 in, 3 out]
        n209 = call "MultiChannel Moving Average Filter PtByPt.vi"("Initialize"=w416, "Number of Averages"=w426, "X"=w393) -> ("Filtered X"=w378:dbl[])  [unwired: 8 in]
        n210 = Array Size(array=w430) -> (size(s)=w431:i32)
        n211 = case shown="\"FOFB Mode\"" w398 {
          tunnel: [T1."Corr. órbita via OPR1" ("Operation Mode (Controller to GUI)") T1."Corr. órbita via FOFB" ("Operation Mode (Controller to GUI)") T1."Medida de Matriz Resposta" ("Operation Mode (Controller to GUI)")] -> w419
          frame "Manual Mode", Default {
          }
          frame "FOFB Mode" {
          }
          frame "RMM Mode" {
          }
        }
        "Operation Mode (Controller to GUI)" <- w419
        n212 = call "MultiChannel Moving Average Filter PtByPt.vi"("Initialize"=w416, "Number of Averages"=u32 100, "X"=w378) -> ("Filtered X"=→"Current Orbit":dbl[])  [unwired: 8 in]
        n213 = feedback #3() -> (w432:dbl[])
        n214 = case shown="1, Default" w431 {
          tunnel: w430 -> [_ w548]
          tunnel: w432 -> [w547 _]
          tunnel: [w547 w548] -> w377
          frame 0 {
          }
          frame 1, Default {
          }
        }
        "Reference Orbit" <- w377
        n215 = feedback-in #3(w377) -> ()
        n216 = Subtract(x=w378, y=w377) -> (x-y=w395:dbl[])
        n217 = feedback #4() -> (w427:u32)  [unwired: 1 in]
        n218 = Equal?(x=w425, y=w427) -> (x = y?=w429:bool)
        n219 = case shown="True" w429 {
          tunnel: w427 -> [w491 _]
          tunnel: [w490 u32 0] -> w428
          tunnel: w415 -> [_ w512]
          tunnel: w414 -> [_ w508]
          tunnel: w395 -> [_ w503]
          tunnel: w413 -> [_ w502]
          frame False {
            n220 = Increment(x=w491) -> (x+1=w490:u32)
          }
          frame True {
            n221 = Split 1D Array(array=w503, index=w502) -> (first subarray=w499:dbl[], second subarray=w501:dbl[])
            n222 = for {
              tunnel: [w546] -> w504 mode=indexing
              tunnel: w499 -> [w544] mode=indexing
              i -> [w545]
              n223 = Bundle(w545, w544) -> (w546:cluster{i32, dbl})  [unwired: 1 in]
            }
            "Horizontal" <- w504
            n224 = for {
              tunnel: w501 -> [w541] mode=indexing
              tunnel: [w543] -> w505 mode=indexing
              i -> [w542]
              n225 = Bundle(w542, w541) -> (w543:cluster{i32, dbl})  [unwired: 1 in]
            }
            "Vertical" <- w505
            n226 = call-poly <vilib>:"RMS.vi"("X"=w499) -> ("rms value"=→"RMS X":dbl)  [unwired: 1 out]
            n227 = call-poly <vilib>:"RMS.vi"("X"=w501) -> ("rms value"=→"RMS Y":dbl)  [unwired: 1 out]
            n228 = Absolute Value(x=w499) -> (abs(x)=w517:dbl[])
            n229 = Absolute Value(x=w501) -> (abs(x)=w513:dbl[])
            n230 = Array Max & Min(array=w517) -> (max value=w493:dbl, max index (indices)=w516:i32, min index (indices)=w498:i32)  [unwired: 1 out]
            n231 = Array Max & Min(array=w513) -> (max value=w492:dbl, max index (indices)=w496:i32, min index (indices)=w497:i32)  [unwired: 1 out]
            n232 = Index Array(array=w512, index #1=w516, index #2=w498) -> (element #1=→"Max X @":string, element #2=→"Min X @":string)
            n233 = Index Array(array=w499, index #1=w516, index #2=w498) -> (element #1=→"Max. X":dbl, element #2=→"Min X":dbl)
            n234 = Index Array(array=w501, index #1=w496, index #2=w497) -> (element #1=→"Max. Y":dbl, element #2=→"Min Y":dbl)
            n235 = Index Array(array=w508, index #1=w496, index #2=w497) -> (element #1=→"MaxY @":string, element #2=→"Min Y @":string)
            n236 = flat-sequence {
              tunnel: "Auto-Scale" -> [w522]
              tunnel: w493 -> [w521]
              tunnel: w492 -> [w520]
              frame #0 {
                n237 = case shown="True" w522 {
                  tunnel: w521 -> [_ w533]
                  tunnel: w520 -> [_ w525]
                  frame False {
                  }
                  frame True {
                    w527 = 10.0 ("y")
                    w523 = 1.2 ("x")
                    w534 = 10.0 ("y")
                    n238 = Multiply(x=w533, y=w534) -> (x*y=w536:dbl)
                    n239 = Multiply(x=w525, y=w527) -> (x*y=w529:dbl)
                    n240 = Round Toward +Infinity(x=w536) -> (ceil(x): smallest int >= x=w535:dbl)
                    n241 = Round Toward +Infinity(x=w529) -> (ceil(x): smallest int >= x=w528:dbl)
                    n242 = Divide(x=w535, y=w534) -> (x/y=w531:dbl)
                    n243 = Divide(x=w528, y=w527) -> (x/y=w526:dbl)
                    n244 = Multiply(x=w523, y=w531) -> (x*y=w530:dbl)
                    n245 = Multiply(x=w523, y=w526) -> (x*y=w524:dbl)
                    n246 = property on="Max Scale X" class="DigNum (strict)"("Value"=w530) -> ()  [unwired: 2 in, 2 out]
                    n247 = property on="Max Scale Y" class="DigNum (strict)"("Value"=w524) -> ()  [unwired: 2 in, 2 out]
                    n248 = property on="Auto-Scale" class="Bool (strict)"("Value"=FALSE) -> ()  [unwired: 2 in, 2 out]
                  }
                }
              }
              frame #1 {
                n249 = Negate(x="Max Scale X") -> (-x=w540:dbl)
                n250 = Negate(x="Max Scale Y") -> (-x=w538:dbl)
                n251 = property on="Horizontal" class="XYGraph (strict)"("YScale.Maximum"="Max Scale X") -> ()  [unwired: 2 in, 2 out]
                n252 = property on="Horizontal" class="XYGraph (strict)"("YScale.Minimum"=w540) -> ()  [unwired: 2 in, 2 out]
                n253 = property on="Vertical" class="XYGraph (strict)"("YScale.Maximum"="Max Scale Y") -> ()  [unwired: 2 in, 2 out]
                n254 = property on="Vertical" class="XYGraph (strict)"("YScale.Minimum"=w538) -> ()  [unwired: 2 in, 2 out]
              }
            }
          }
        }
        n255 = feedback-in #4(w428) -> ()
        n256 = Seconds To Date/Time(time stamp (now)=w390) -> (date time rec=w392:T25)  [unwired: 1 in]
        n257 = Date/Time To Seconds(1:TRUE ("is UTC (F)"), 2:w392) -> (0:w389:timestamp)
        n258 = To Double Precision Float(number=w389) -> (double precision float=w388:dbl)
        n259 = Build Array (concatenate)(w411, w412) -> (w396:dbl[])
        n260 = Bundle By Name(cluster=w409, "Timestamp"=w390, "Sample"=w395) -> (w397:T22)
        n261 = Lossy Enqueue Element(queue=w420, element=w397) -> ()  [unwired: 1 in, 4 out]
        n262 = Lossy Enqueue Element(queue=w406, element=w397) -> ()  [unwired: 1 in, 4 out]
        n263 = Bundle By Name(cluster=T9 {"Timestamp"=timestamp(0 s since 1904-01-01), "Diagnostics Data"={"Time-Critical Loop Missed Iterations"=0, "Time-Critical Loop Execution Time (usec)"=0, "FA Buffer Usage"=0, "Available Memory (bytes)"=0, "CPU Loads Array"=[]}} ("Diagnostics  Sample"), "Diagnostics Data"=w399, "Timestamp"=w390) -> (w408:T9)
        n264 = Lossy Enqueue Element(queue=w405, element=w397) -> ()  [unwired: 1 in, 4 out]
        n265 = Bundle By Name(cluster=w409, "Sample"=w396, "Timestamp"=w390) -> (w410:T22)
        n266 = disable-structure shown="Disabled" {
          disable-tunnel: w396 -> [w477 _]
          disable-tunnel: w394 -> [w476 _]
          disable-tunnel: w393 -> [w475 _]
          disable-tunnel: w388 -> [w474 _]
          disable-tunnel: w387 -> [w471 _]
          disable-tunnel: w385 -> [w470 _]
          disable-tunnel: [w467 _] -> w382
          disable-tunnel: [w466 _] -> w381
          disable-tunnel: w380 -> [w465 _]
          disable-tunnel: w379 -> [w462 _]
          frame Disabled {
            n267 = Build Array (concatenate)(w474, w475, w477) -> (w472:dbl[])
            n268 = TDMS Write(0:w471, 1:enum16{"decimated", "interleaved"}."interleaved" ("data layout (0:decimated)"), 5:"FOFB BPM and PS Monitoring Data" ("group name in (Untitled)"), 7:w476, 9:w472, 11:w470) -> (4:w468:refnum<k34>, 15:w469:errorcluster)  [unwired: 2 out]
            n269 = Less Or Equal To 0?(x=w465) -> (x <= 0?=w464:bool)
            n270 = Compound Arithmetic op=OR(w464, w462) -> (w463:bool)
            n271 = case shown="True" w463 {
              tunnel: w469 -> [w479 w483]
              tunnel: w468 -> [w480 w482]
              tunnel: [w480 _] -> w467
              tunnel: [w479 w481] -> w466
              frame False {
              }
              frame True {
                n272 = TDMS Close(8:w483, 11:w482) -> (0:w481:errorcluster)  [unwired: 1 out]
              }
            }
          }
          frame Enabled {
          }
        }
        n273 = Lossy Enqueue Element(queue=w404, element=w410) -> ()  [unwired: 1 in, 4 out]
        n274 = Lossy Enqueue Element(queue=w403, element=w410) -> ()  [unwired: 1 in, 4 out]
        n275 = Lossy Enqueue Element(queue=w402, element=w410) -> ()  [unwired: 1 in, 4 out]
        n276 = flat-sequence {
          tunnel: [w489] -> w424
          tunnel: w421 -> [w489]
          tunnel: w423 -> [w488]
          tunnel: [w487] -> w379
          frame #0 {
            n277 = Wait on Notification(notifier=w488, timeout in ms (-1)=0) -> (notification=w487:bool)  [unwired: 2 in, 3 out]
          }
        }
        n278 = Lossy Enqueue Element(queue=w401, element=w408) -> ()  [unwired: 1 in, 4 out]
        n279 = node-c288() -> ()  [unwired: 1 in, 1 out]
      }
      n280 = node-c288(w80) -> ()  [unwired: 1 out]
      n281 = Close Reference(reference=w60) -> (error out=w58:errorcluster)  [unwired: 1 in]
      n282 = node-c288(w82) -> ()  [unwired: 1 out]
      n283 = Merge Errors(w58, w73, w70, w71, w26, w33, w72) -> (w59:errorcluster)
      n284 = call "GUI Close Synchronization Objects.vi"("error in (no error)"=w59, "FOFB GUI"=w11) -> ("error out"=→"error out":errorcluster)  [unwired: 9 in]
    }
    frame True {
    }
  }
